vi "Begin.vi"() -> (0 "error out":errorcluster)   [LabVIEW 2013]
doc: "Called before other user functions, this VI is expected to open initial I/O refnums, load in file data, and do all program initialization. Notice that the <B>error out</B> terminal is simply used for data flow. Wiring it to other structures or subVIs ensures that this VI runs first."
uses:
  <vilib>/Rock Robotics/SystemInterfaces/AI/FPGA_AIGyroChannel.ctl
  <vilib>/Rock Robotics/SystemInterfaces/Typedef/FPGA_TypedefAnalogModuleForGyro.ctl
  <vilib>/Rock Robotics/SystemInterfaces/DIO/FPGA_DIOPWMChannel.ctl
  <vilib>/Rock Robotics/WPI/SafetyOutput/WPI_SafetyOutputConfigMenu.ctl
  <vilib>/Rock Robotics/WPI/DriverStation/WPI_DriverStationRobotMode2.ctl
  <vilib>/Rock Robotics/WPI/Joystick/WPI_JoystickDeviceEnum.ctl
  <vilib>/Rock Robotics/WPI/RobotDrive/WPI_RobotDriveOpen2MotorWithJaguar.vi
  Robot Global Data.vi
panel:
  in  "Analog Module":T1
  in  "Gain (VoltsPerDegree/Second)":dbl=0.0125
  in  "Channel":T2
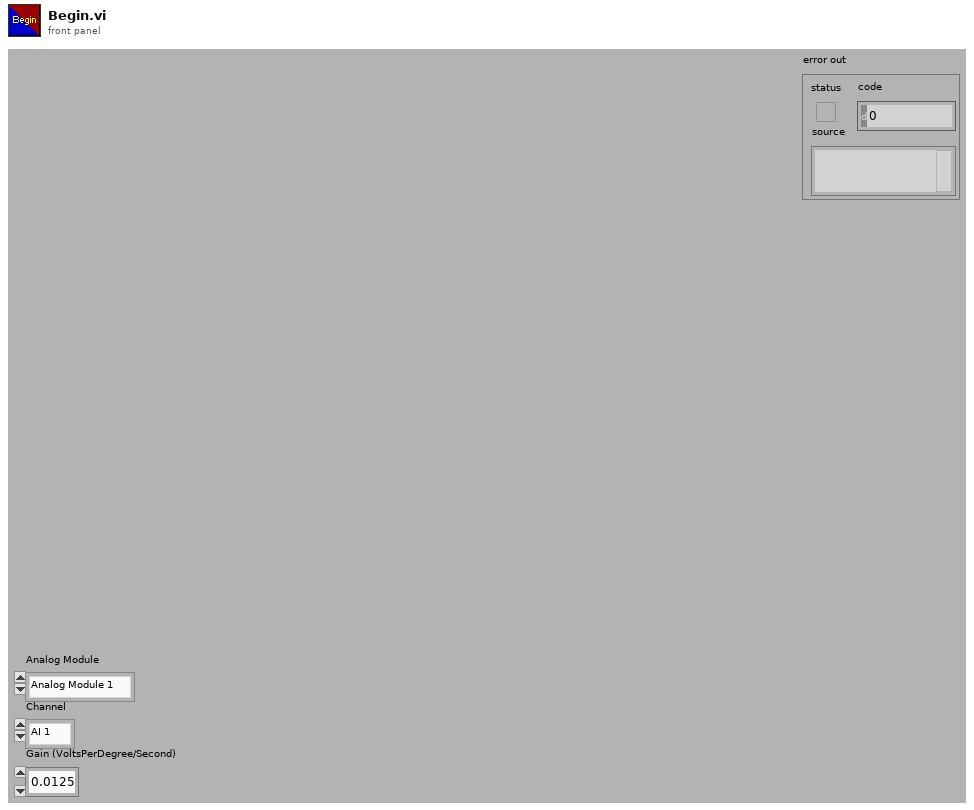
[diagram p1: front panel]
types:
  T1 = typedef "FPGA_TypedefAnalogModuleForGyro.ctl" = enum16{"Analog Module 1"}
  T2 = typedef "FPGA_AIGyroChannel.ctl" = enum8{"AI 1", "AI 2", "Invalid"}
  T3 = typedef "WPI_JoystickDeviceEnum.ctl" = enum16{"USB 1", "USB 2", "USB 3", "USB 4", "Kinect 1", "Kinect 2"}
  T4 = typedef "WPI_DriverStationRobotMode2.ctl" = enum16{"Autonomous Disabled", "Autonomous Enabled", "Teleop Disabled", "Teleop Enabled", "Timeout", "Finish", "Test Disabled", "Test Enabled"}
  T5 = typedef "WPI_SafetyOutputConfigMenu.ctl" = enum16{"Enable", "Disable"}
  T6 = typedef "FPGA_DIOPWMChannel.ctl" = enum8{"PWM 1", "PWM 2", "PWM 3", "PWM 4", "PWM 5", "PWM 6", "PWM 7", "PWM 8", "PWM 9", "PWM 10", "Invalid"}
  T7 = typedef "WPI_GyroDevRef.ctl" = cluster{"DevStatus":errorcluster, "Analog Module":T8, "Analog Channel":T9, "Offset":dbl, "Gain (VoltsPerDegree/Second)":dbl}
  T8 = typedef "FPGA_TypedefAnalogModule.ctl" = enum16{"Analog Module 1", "Analog Module 2"}
  T9 = typedef "FPGA_AIChannel.ctl" = enum8{"AI 1", "AI 2", "AI 3", "AI 4", "AI 5", "AI 6", "AI 7", "AI 8", "Invalid"}
  T10 = typedef "WPI_JoystickDevRef.ctl" = cluster{"Device":T3}
  T11 = typedef "WPI_RobotDriveDevRef.ctl" = cluster{"DevStatus":errorcluster, "Motors[]":T12[], "Square Inputs":bool, "Max Output":dbl, "Isochronous":bool}
  T12 = typedef "WPI_MotorControlDeviceRef.ctl" = cluster{"DeviceStatus":errorcluster, "Type":enum16{"PWM", "CAN"}, "PWM":cluster{"Digital Module":T13, "PWM Channel":T6, "DeadBand":T14}, "CAN":cluster{"Device Number":u8, "Control Mode":T15, "Semaphore":T16, "Max Vout":dbl}, "Invert":bool, "TransformRef":T17, "InvTransformRef":T17}
  T13 = typedef "FPGA_TypedefDigitalModule.ctl" = enum16{"Digital Module 1", "Digital Module 2"}
  T14 = typedef "WPI_PWMDeadband.ctl" = cluster{"Name":string, "maxPositivePwm":i32, "minPositivePwm":i32, "centerPwm":i32, "maxNegativePwm":i32, "minNegativePwm":i32, "angularRange":u16}
  T15 = typedef "WPI_CANJaguar_ControlMode.ctl" = enum8{"Percent VBus", "Current", "Speed", "Position", "Voltage"}
  T16 = typedef "Semaphore RefNum" = refnum<k1>
  T17 = typedef "WPI_PWMTransform_ConPane.ctl" = refnum<vi>
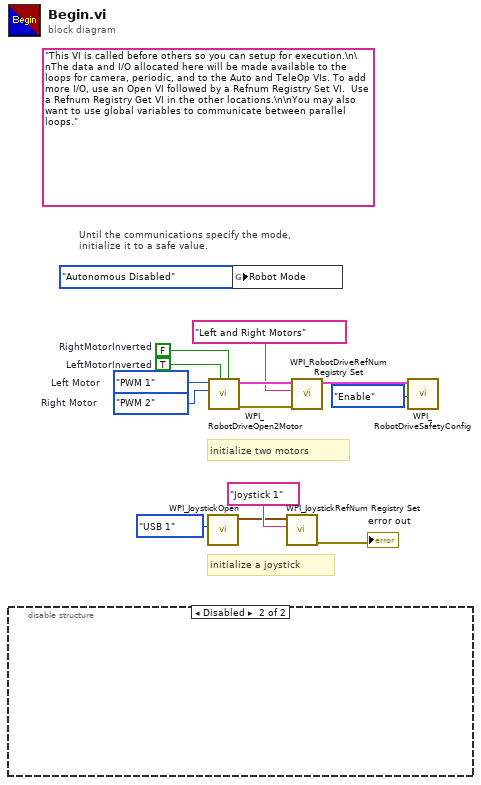
[diagram p0: block diagram]
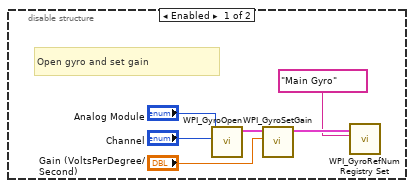
[diagram p2: hidden frame]
diagram:
  (unwired) "This VI is called before others so you can setup for execution.\n\nThe data and I/O allocated here will be made available to the loops for camera, periodic, and to the Auto and TeleOp VIs. To add more I/O, use an Open VI followed by a Refnum Registry Set VI.  Use a Refnum Registry Get VI in the other locations.\n\nYou may also want to use global variables to communicate between parallel loops."
  w8 = FPGA_DIOPWMChannel."PWM 2"  # Right Motor
  w9 = FPGA_DIOPWMChannel."PWM 1"  # Left Motor
  w13 = TRUE  # LeftMotorInverted
  w14 = FALSE  # RightMotorInverted
  # "initialize a joystick"
  # "Until the communications specify the mode,\ninitialize it to a safe value."
  # "initialize two motors"
  n1 = disable-structure shown="Disabled" {
    frame Enabled {
      # "Open gyro and set gain"
      n2 = call <vilib>:"WPI_GyroOpen.vi"("Analog Channel"="Channel", "Analog Module (Module 1)"="Analog Module") -> ("GyroDevRef"=w16:T7)  [unwired: 4 in, 5 out]
      n3 = call <vilib>:"WPI_GyroSetGain.vi"("Gain (VoltsPerDegree/Second)"="Gain (VoltsPerDegree/Second)", "GyroDevRef"=w16) -> ("GyroDevRef"=w20:T7)  [unwired: 1 in, 8 out]
      n4 = call <vilib>:"WPI_GyroRefNum Registry Set.vi"("refnum name"="Main Gyro", "GyroDevRef"=w20) -> ()  [unwired: 8 in, 2 out]
    }
    frame Disabled {
    }
  }
  n5 = call <vilib>:"WPI_JoystickOpen.vi"("JoystickDevice"=WPI_JoystickDeviceEnum."USB 1") -> ("JoystickDevRef"=w3:T10)  [unwired: 10 in]
  n6 = call-poly <vilib>:"WPI_RobotDriveOpen2Motor.vi"("Right Motor Inverted"=w14, "Left Motor Inverted"=w13, "Right Motor"=w8, "Left Motor"=w9) -> ("error out"=w10:errorcluster, "RobotDriveDevRef"=w12:T11)  [unwired: 1 in, 5 out]
  n7 = global write "Robot Global Data.vi" "Robot Mode"(WPI_DriverStationRobotMode2."Autonomous Disabled" ("Robot Mode")) -> ()
  n8 = call <vilib>:"WPI_JoystickRefNum Registry Set.vi"("refnum name"="Joystick 1", "JoystickDevRef"=w3) -> ("error out"=→"error out":errorcluster)  [unwired: 8 in, 1 out]
  n9 = call <vilib>:"WPI_RobotDriveRefNum Registry Set.vi"("error in (no error)"=w10, "refnum name"="Left and Right Motors", "RobotDriveDevRef"=w12) -> ("RobotDriveDevRef"=w7:T11)  [unwired: 8 out]
  n10 = call <vilib>:"WPI_RobotDriveSafetyConfig.vi"("mode"=WPI_SafetyOutputConfigMenu."Enable", "RobotDriveDevRef"=w7) -> ()  [unwired: 8 in, 2 out]
